vi "Initialize.vi"(8 "Error In":errorcluster) -> (0 "Error Out":errorcluster)   [LabVIEW 2023, in "QSM - Main.lvlib"]
doc: "This VI sends the Initialize message to the Queued Message Handler template."
uses:
  QSM - Main.lvlib
  SubVIs/Enqueue Message (Single).vi
  Controls/Message Queue Element Position.ctl
  Controls/State Machine Message.ctl
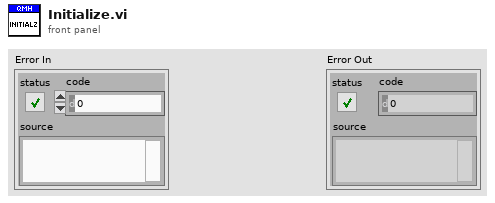
[diagram p1: front panel]
types:
  T1 = typedef "QSM - Main.lvlib/State Machine Message.ctl" = enum16{"Initialize", "Operator Signon", "Editor", "Security", "Select Tube", "Select Sched", "View Sched", "View IO/DOCS", "New Gx Val", "View LIMITS", "View ALARMS", "Start Step Change", "New Serial Number", "RUN Initiated", "RESET Initiated", "PLC Step Change", "PROC OK CHECK", "PROC NOK", "ALARM CHECK", "ALARM ACTIVE", "CHECKS", "BIAS ZER", "DIFF ZER", "DIFF TOGGLE", "Handle Error", "Exit"}
  T2 = typedef "QSM - Main.lvlib/Message Queue Element Position.ctl" = enum16{"Front", "Back"}
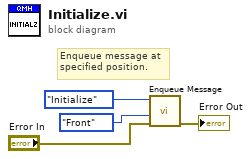
[diagram p0: block diagram]
diagram:
  # "Enqueue message at\nspecified position."
  n1 = call-poly "Enqueue Message.vi"("Error In"="Error In", "Message Position"=Message_Queue_Element_Position."Front", "State Machine Message"=State_Machine_Message."Initialize") -> ("Error Out"=→"Error Out":errorcluster)  [unwired: 8 in]
